vi "Matches.vi"(8 "error in (no error)":errorcluster, 10 "Actual":variant, 11 "Collection Is Equivalent in":refnum<class "Collection Is Equivalent.lvclass">) -> (0 "error out":errorcluster, 2 "Result":bool, 3 "Collection Is Equivalent out":refnum<class "Collection Is Equivalent.lvclass">)   [LabVIEW 2017, in "Transparent Assertions.lvlib" / "Collection Is Equivalent.lvclass"]
doc: "Evaluates the constraint for <B>Actual</B>. Returns true if the constraint is met."
uses:
  Collection Is Equivalent.lvclass
  Collection Is Equivalent.lvclass/Collection Is Equivalent.ctl
  Transparent Assertions.lvlib
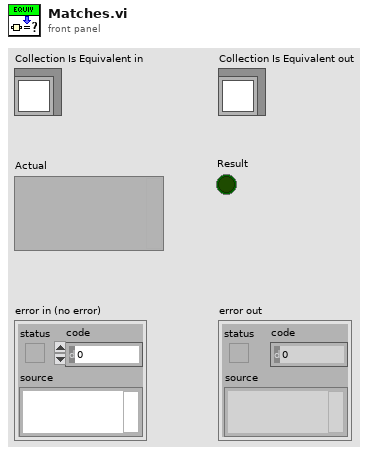
[diagram p1: front panel]
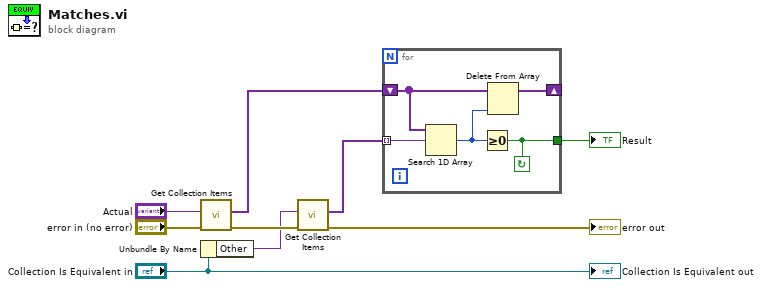
[diagram p0: block diagram]
diagram:
  n1 = call "Get Collection Items.vi"("error in (no error)"="error in (no error)", "Collection"="Actual") -> ("error out"=w7:errorcluster, "Items"=w4:variant[])  [unwired: 8 in]
  n2 = Unbundle By Name("Collection Is Equivalent in") -> ("Other"=w5:variant)
  n3 = call "Get Collection Items.vi"("error in (no error)"=w7, "Collection"=w5) -> ("error out"=→"error out":errorcluster, "Items"=w3:variant[])  [unwired: 8 in]
  n4 = for {
    tunnel: w3 -> [w14] mode=indexing
    shift-right: [w12] -> _
    shift-left: w4 -> [w13]
    tunnel: [w10] -> w1
    stop <- w10 continue-if-true
    n5 = Search 1D Array(1D array=w13, element=w14) -> (index of element=w11:i32)  [unwired: 1 in]
    n6 = Greater Or Equal To 0?(x=w11) -> (x >= 0?=w10:bool)
    n7 = Delete From Array(array=w13, index=w11) -> (array with subset deleted=w12:variant[])  [unwired: 1 in, 1 out]
  }
  "Result" <- w1
  "Collection Is Equivalent out" <- "Collection Is Equivalent in"
